vi "generate string.vi"(11 "base string":string) -> (3 "json string":string)   [LabVIEW 2013, in "json generator.lvlib"]
uses:
  json generator.lvlib
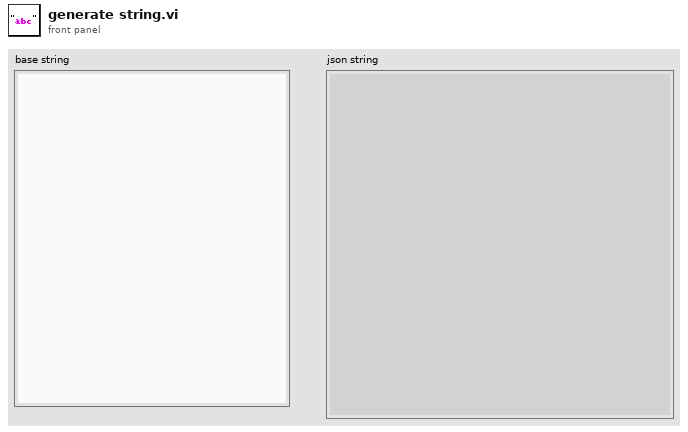
[diagram p1: front panel]
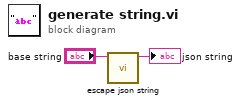
[diagram p0: block diagram]
diagram:
  n1 = call "escape json string.vi"("base string"="base string") -> ("String out"=→"json string":string)  [unwired: 10 in]
